vi "SeCrTs-Seq Display.vi"(8 "error in":errorcluster, 9 "Seq Monitor":string[](array[string])) -> (0 "error out":errorcluster, 1 "out":string)   [LabVIEW 2022 SP3]
uses:
  7d550175-5455-4006-8214-fd52ac005701.vi
panel:
  out "changed or first call?":bool
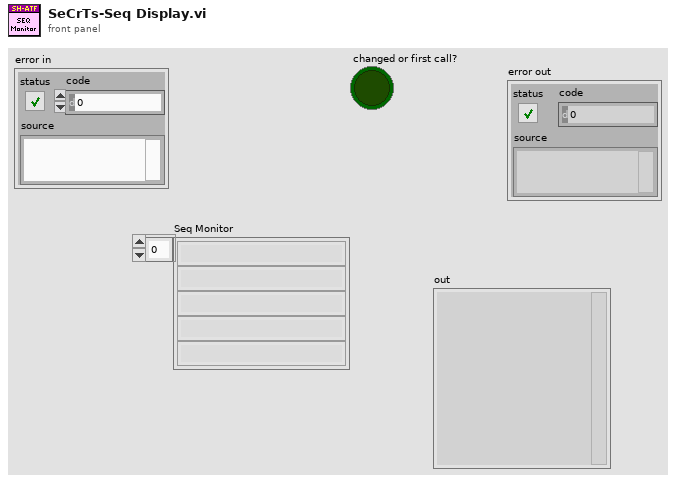
[diagram p1: front panel]
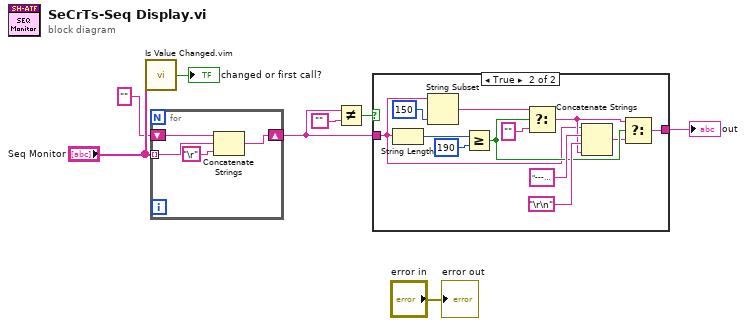
[diagram p0: block diagram]
diagram:
  n1 = call "Is Value Changed.vim"("value"="Seq Monitor") -> ("changed or first call?"=→"changed or first call?":bool)
  n2 = for {
    tunnel: "Seq Monitor" -> [w12] mode=indexing
    shift-right: [w11] -> w3
    shift-left: "" -> [w9]
    n3 = Concatenate Strings(w9, w12, "\r") -> (w11:string)
  }
  n4 = Not Equal?(x=w3, y="") -> (x != y?=w4:bool)
  n5 = case shown="True" w4 {
    tunnel: w3 -> [_ w14]
    tunnel: [_ w16] -> w7
    frame False {
    }
    frame True {
      n6 = String Length(string=w14) -> (length=w24:i32)
      n7 = String Subset(string=w14, length (rest)=150 ("length (rest)")) -> (substring=w21:string)  [unwired: 1 in]
      n8 = Greater Or Equal?(x=w24, y=190) -> (x >= y?=w18:bool)
      n9 = Select(t=w21, s=w18, f="") -> (s? t:f=w17:string)
      n10 = Concatenate Strings(w14, "------------" ("string"), "\r\n", w17) -> (w15:string)
      n11 = Select(t=w17, s=w18, f=w15) -> (s? t:f=w16:string)
    }
  }
  "out" <- w7
  "error out" <- "error in"
